vi "FindUserAppFolder.vi"(8 "error in":errorcluster) -> (0 "error out":errorcluster, 3 "UserPath":path)   [LabVIEW 2010]
uses:
  <vilib>/registry/registry.llb/Registry RtKey.ctl
  <vilib>/registry/registry.llb/Read Registry Value Simple STR.vi
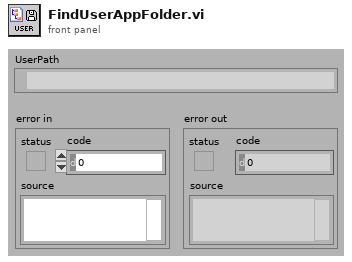
[diagram p1: front panel]
types:
  T1 = typedef "Registry RtKey.ctl" = enum32{"HKEY_CLASSES_ROOT", "HKEY_CURRENT_USER", "HKEY_LOCAL_MACHINE", "HKEY_USERS", "HKEY_PERFORMANCE_DATA", "HKEY_CURRENT_CONFIG", "HKEY_DYN_DATA"}
  T2 = typedef "Registry refnum.ctl" = refnum<k1>
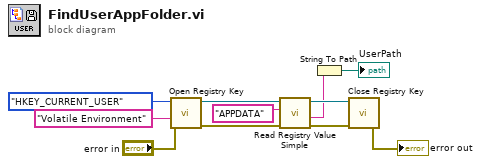
[diagram p0: block diagram]
diagram:
  n1 = call <vilib>:"Open Registry Key.vi"("error in (no error)"="error in", "subkey"="Volatile Environment", "root key (HKEY_LOCAL_MACHINE)"=Registry_RtKey."HKEY_CURRENT_USER") -> ("error out"=w6:errorcluster, "refnum out"=w8:T2)  [unwired: 7 in]
  n2 = call-poly <vilib>:"Read Registry Value Simple.vi"("error in (no error)"=w6, "value"="APPDATA", "refnum"=w8) -> ("error out"=w5:errorcluster, "String/Binary data"=w4:string, "refnum out"=w7:T2)  [unwired: 3 in, 1 out]
  n3 = String To Path(string=w4) -> (path=→"UserPath":path)
  n4 = call <vilib>:"Close Registry Key.vi"("error in (no error)"=w5, "refnum"=w7) -> ("error out"=→"error out":errorcluster)  [unwired: 5 in]
